vi "Is Terminate.vi"(5 "Stop Refnum":refnum<vi>, 6 "error in":errorcluster, 8 "code (-1)":i32=-1) -> (0 "error out":errorcluster, 2 "terminated":bool)   [LabVIEW 2010]
doc: "If the input error status is FALSE (no error) and the STOP control refnum value is TRUE, then this function puts the message \"Terminated by user at x:xx AM/PM.\" with the current time in the error message cluster and sets the error status to TRUE. \n\nIf the input error status is TRUE (error) the existing error cluster is unchanged."
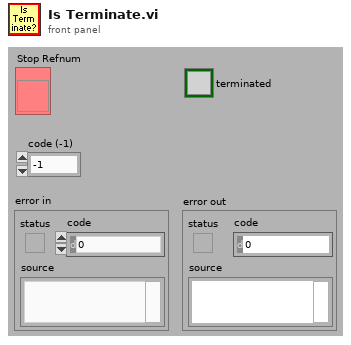
[diagram p1: front panel]
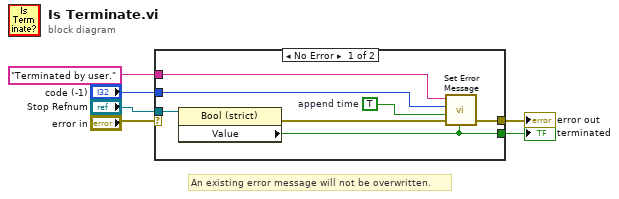
[diagram p0: block diagram]
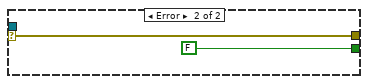
[diagram p2: hidden frame]
diagram:
  # "An existing error message will not be overwritten."
  n1 = case shown="No Error" "error in" {
    selector: "error in" -> [_ w15]
    tunnel: "Stop Refnum" -> [w13 _]
    tunnel: [w12 w15] -> w6
    tunnel: "Terminated by user." ("Message") -> [w11 _]
    tunnel: [w8 FALSE] -> w2
    tunnel: "code (-1)" -> [w9 _]
    frame No Error {
      w7 = TRUE  # append time
      n2 = property class="Bool (strict)"(reference=w13) -> (error out=w10:errorcluster, "Value"=w8:bool)  [unwired: 1 in, 1 out]
      n3 = call "Set Error Message.vi"("enable (T)"=w8, "error in"=w10, "append time (F)"=w7, "code (-1)"=w9, "message"=w11) -> ("error out"=w12:errorcluster)  [unwired: 3 in]
    }
    frame Error {
    }
  }
  "error out" <- w6
  "terminated" <- w2
